vi "ALP_FLUT_Mode_18bit_4395_.vi"(8 "error in (no error)":errorcluster, 10 "SequenceId in":u32, 11 "DeviceId in":u32) -> (0 "error out":errorcluster, 1 "SequenceId out":u32, 2 "DeviceId out":u32)   [LabVIEW 2020]
uses:
  <vilib>/Utility/error.llb/Error Cluster From Error Code.vi
  <userlib>/alp4395/alp4395.dll
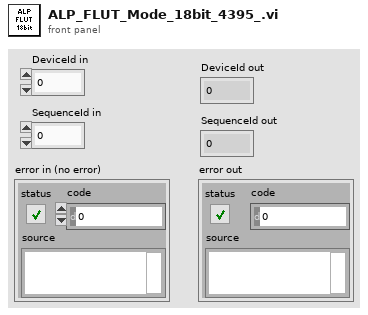
[diagram p1: front panel]
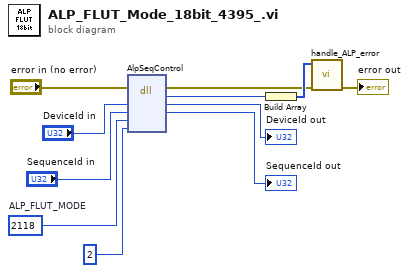
[diagram p0: block diagram]
diagram:
  w6 = 2118  # ALP_FLUT_MODE
  n1 = dll-call lib="C:/Program Files (x86)/National Instruments/LabVIEW 2020/user.lib/alp4395/alp4395.dll" fn="AlpSeqControl"(error in="error in (no error)", "DeviceId"="DeviceId in", "SequenceId"="SequenceId in", "ControlType"=w6, "ControlValue"=2) -> (error out=w2:errorcluster, "return type"=w4:i32, "DeviceId"=→"DeviceId out":u32, "SequenceId"=→"SequenceId out":u32)  [unwired: 4 in, 1 out]
  n2 = Build Array(w4) -> (w3:i32[])
  n3 = call "handle_ALP_error.vi"("error in"=w2, "Return Codes"=w3) -> ("error out"=→"error out":errorcluster)  [unwired: 9 in]
